vi "Elements.vi"() -> (1 "Elements available":T1(array[cluster]))   [LabVIEW 2009]
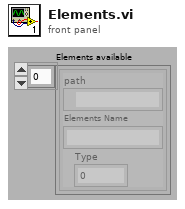
[diagram p1: front panel]
types:
  T1 = cluster{"path":path, "Elements Name":string, "Type":i32}[]
  T2 = cluster{"path":path, "Button Name":string, "Type":i32}
  T3 = cluster{"path":path, "Elements Name":string, "Type":i32}
  T4 = cluster{"path":path, "Button Name":string, "Type":i32}[]
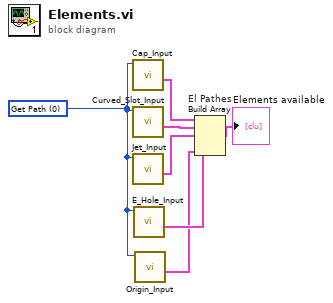
[diagram p0: block diagram]
diagram:
  w2 = u16 0 items=["Get Path", "Make Layout"] ("Outputmode")
  n1 = call "Cap_Input.vi"("Outputmode"=w2) -> ("Init Cluster"=w6:T2)  [unwired: 3 in, 3 out]
  n2 = call "Curved_Slot_Input.vi"("Outputmode"=w2) -> ("Init Cluster"=w4:T2)  [unwired: 3 in, 3 out]
  n3 = call "Jet_Input.vi"("Outputmode"=w2) -> ("Init Cluster"=w5:T3)  [unwired: 3 in, 3 out]
  n4 = call "E_Hole_Input.vi"("Outputmode"=w2) -> ("Init Cluster"=w3:T2)  [unwired: 3 in, 3 out]
  n5 = call "Origin_Input.vi"("Outputmode"=w2) -> ("Init Cluster"=w1:T2)  [unwired: 3 in, 3 out]
  n6 = Build Array "El Pathes"(w6, w4, w5, w3, w1) -> (→"Elements available":T4)
